vi "Database Message Loop.vi"(8 "error in":errorcluster, 10 "Message Queues":T1, 11 "Clust Refnum":refnum<vi>) -> (0 "error out":errorcluster)   [LabVIEW 2025]
doc: "This example allows you to perform several tasks on the specified table in a database named LabVIEW.mdb located in the LabVIEW examples>>database directory.\n\nThis VI is running when you open it. Select one of the tabs and enter the appropriate data. Press the Go button to complete the displayed tab option.\n\nAutomatic - This option inserts a new record into the specified table. The record is specified by a cluster containing the correct number of elements and of the data types defined by the specified table. \n\nSQL Query - This option performs the specified SQL query.\n\nParameterized SQL Query - This option performs the specified SQL query as a parameterized SQL Query. This method is faster and more efficient than directly executing an SQL query because it sets up all the parameters prior to doing the command."
uses:
  support/Message Queue/All Message Queues.ctl
  support/Message Queue/Message Cluster.ctl
  controls/Design_Results.ctl
  <vilib>/drjdpowell/SQLite Library/SQL Statement/SQL Statement.lvclass
  <vilib>/drjdpowell/SQLite Library/SQL Connection/Connection.lvclass
  <vilib>/drjdpowell/SQLite Library/SQL Statement/SQL Statement.lvclass/SQL Statement.ctl
  <vilib>/drjdpowell/SQLite Library/SQL Connection/Open (string).vi
  <vilib>/drjdpowell/SQLite Library/SQL Statement/Bind Timestamp (Local Time Offset).vi
  <vilib>/drjdpowell/SQLite Library/SQL Statement/Bind Real.vi
  <vilib>/drjdpowell/SQLite Library/SQL Statement/Bind Text.vi
  <vilib>/drjdpowell/SQLite Library/SQL Statement/Bind Integer.vi
  <vilib>/drjdpowell/SQLite Library/SQL Statement/Step.vi
  <vilib>/JDP Science/JDP Science Common Utilities/Timestamp/Timestamp to Text.vi
  <vilib>/drjdpowell/SQLite Library/SQL Statement/Bind UTF-8 Text.vi
  <vilib>/Utility/error.llb/Error Cluster From Error Code.vi
  <vilib>/drjdpowell/SQLite Library/SQL Connection/Execute SQL (No results).vi
  <vilib>/drjdpowell/SQLite Library/SQL Statement/Error Message.vi
  <vilib>/ErrorRing/Error Ring.xnode
  support/Message Queue/Message Queue.lvlib
  <vilib>/drjdpowell/SQLite Library/SQLite.lvlib
panel:
  # "Simulator Fit"
  # "Empirical Fit"
  # "="
  # "P"
  # "* X"
  # "P"
  # "="
  # "* X"
  # "drop"
  # "drop"
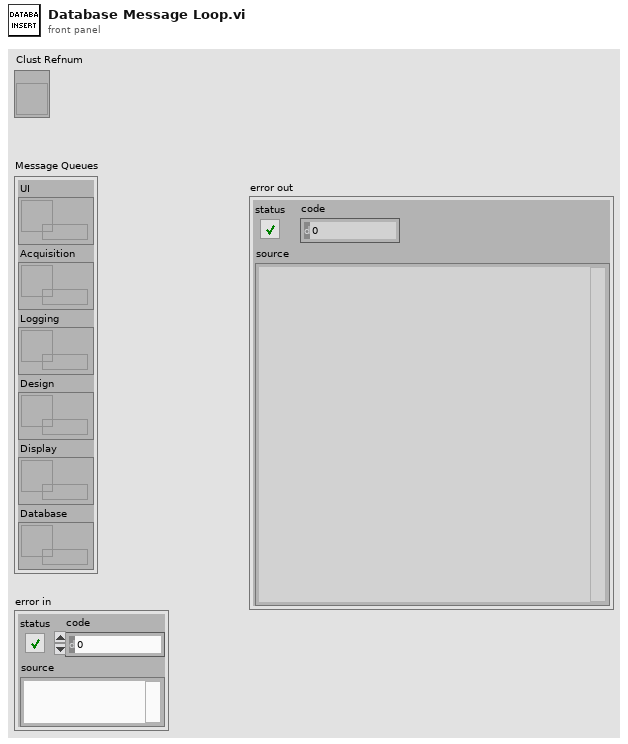
[diagram p1: front panel]
types:
  T1 = typedef "Message Queue.lvlib/All Message Queues.ctl" = cluster{"UI":refnum<queue>, "Acquisition":refnum<queue>, "Logging":refnum<queue>, "Design":refnum<queue>, "Display":refnum<queue>, "Database":refnum<queue>}
  T2 = typedef "Results.ctl" = cluster{"Design Results":cluster{"Model Validation: Simulated vs. Empirical Airflow Data":cluster{dbl[], dbl[]}[], "Amplitude - Empirical":string, "Power - Empirical":string, "Amplitude - Sim":string, "Power - Sim":string, "Flow Type":u32, "Optimized Inlet \nOrifice Diameter (in)":dbl, "Flow Type Name":string}}
  T3 = cluster{"Model Validation: Simulated vs. Empirical Airflow Data[0]":cluster{dbl[], dbl[]}, "Model Validation: Simulated vs. Empirical Airflow Data[1]":cluster{dbl[], dbl[]}, "Model Validation: Simulated vs. Empirical Airflow Data[2]":cluster{dbl[], dbl[]}, "Model Validation: Simulated vs. Empirical Airflow Data[3]":cluster{dbl[], dbl[]}, "Model Validation: Simulated vs. Empirical Airflow Data[4]":cluster{dbl[], dbl[]}, "Model Validation: Simulated vs. Empirical Airflow Data[5]":cluster{dbl[], dbl[]}, "Model Validation: Simulated vs. Empirical Airflow Data[6]":cluster{dbl[], dbl[]}, "Model Validation: Simulated vs. Empirical Airflow Data[7]":cluster{dbl[], dbl[]}, "Model Validation: Simulated vs. Empirical Airflow Data[8]":cluster{dbl[], dbl[]}}
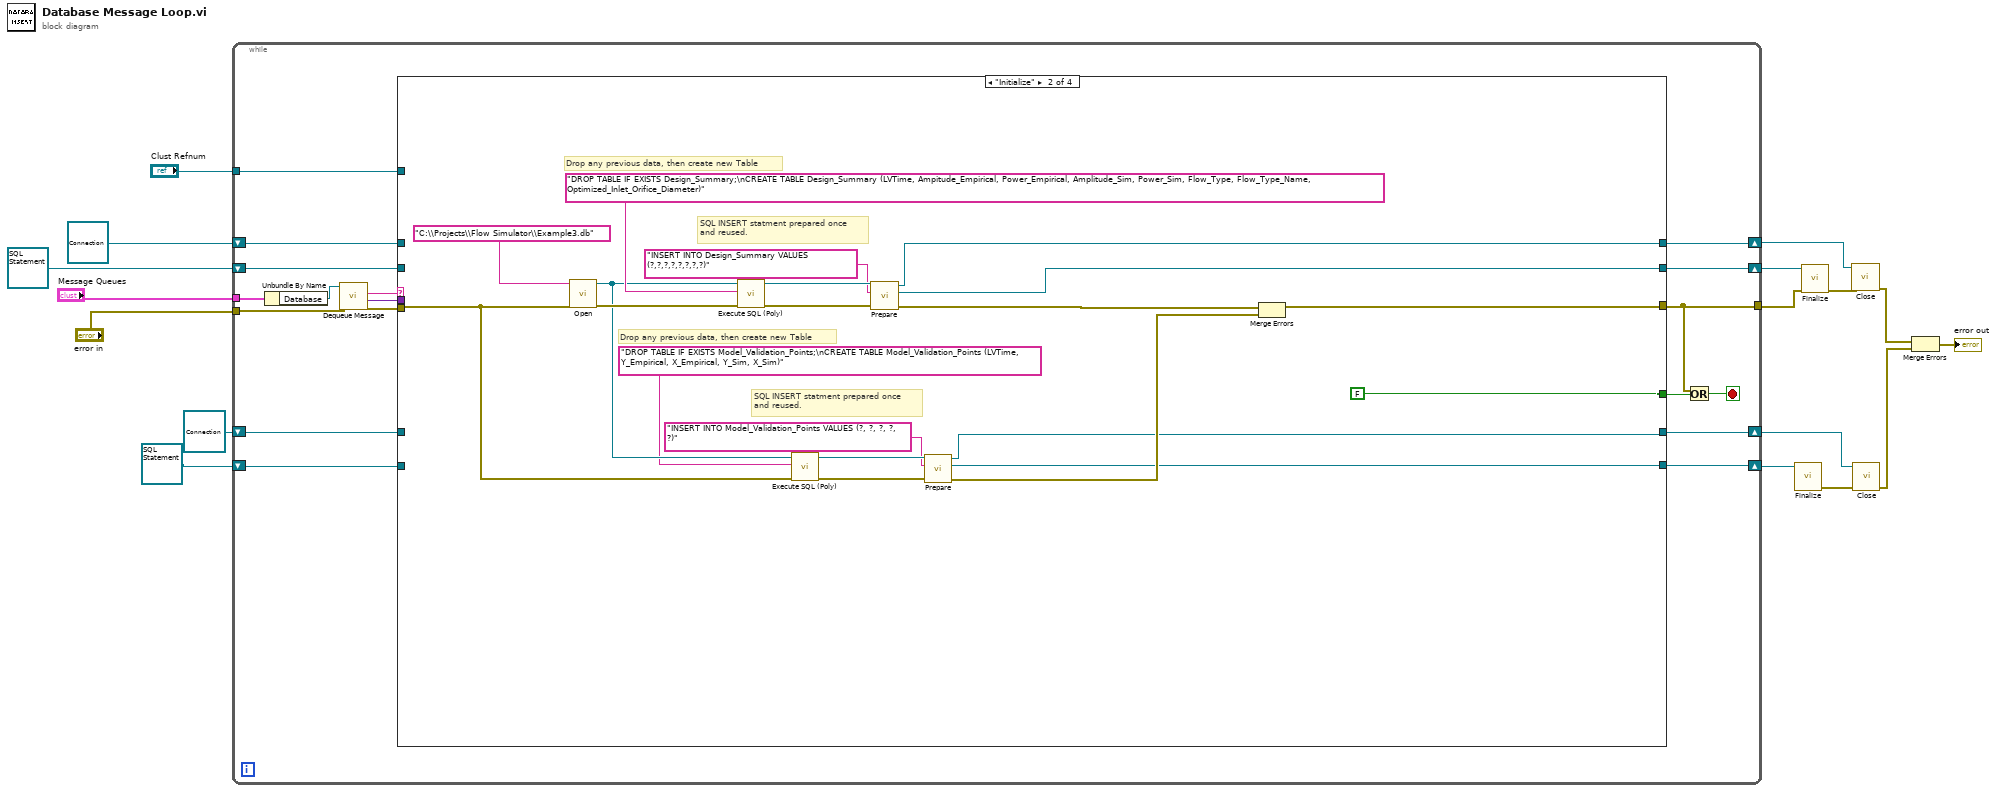
[diagram p0: block diagram]
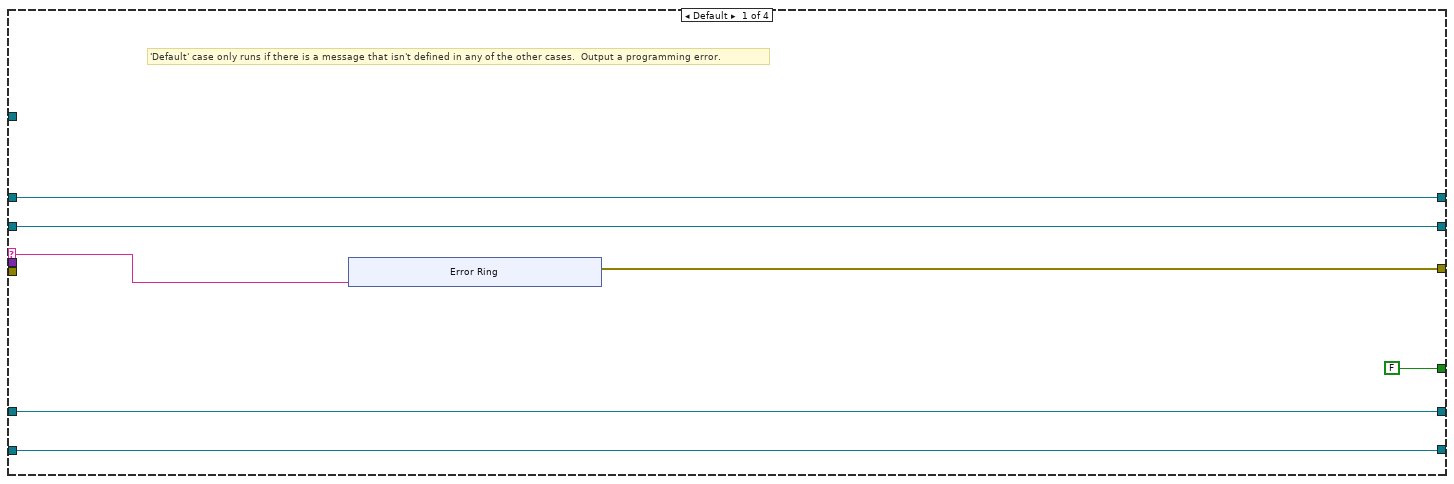
[diagram p2: hidden frame]
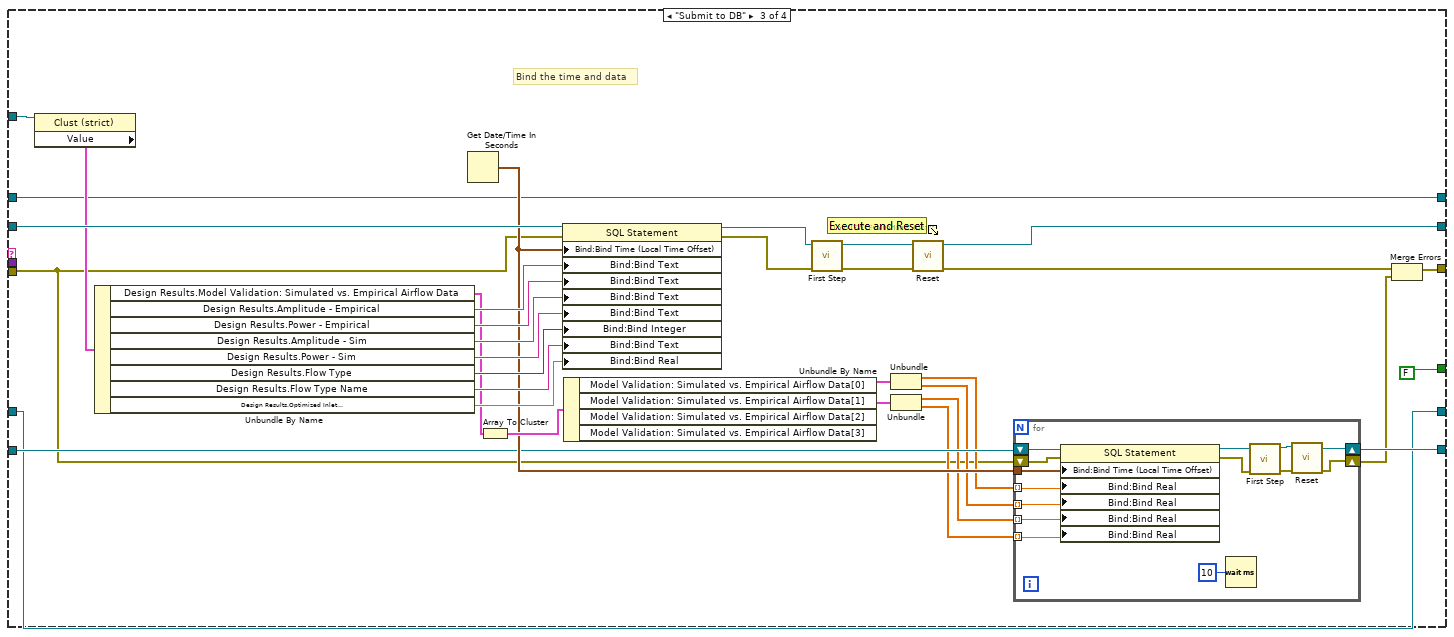
[diagram p3: hidden frame]
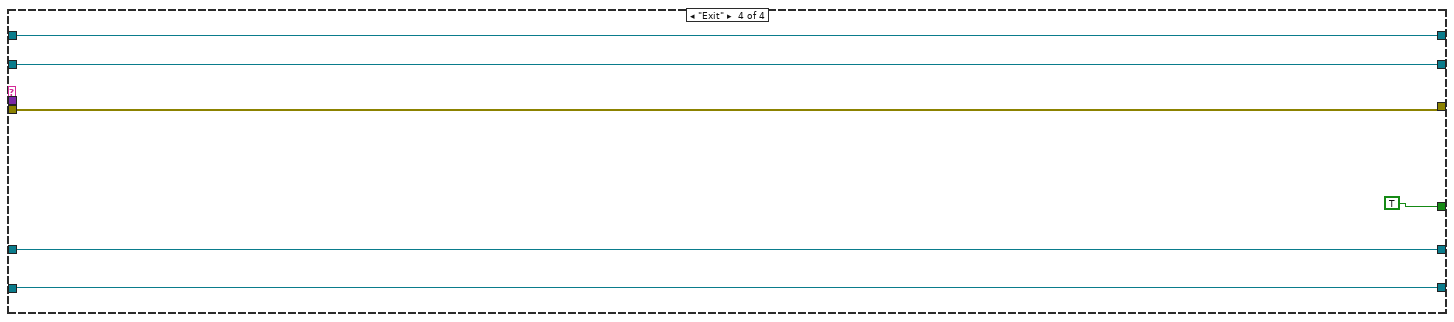
[diagram p4: hidden frame]
diagram:
  n1 = while {
    tunnel: "Message Queues" -> [w34]
    tunnel: [w30] -> w8
    tunnel: "error in" -> [w31]
    shift-right: [w26] -> w9
    shift-left: refnum<class "SQL Statement.lvclass"> refnum ("SQL Statement") -> [w27]
    shift-right: [w23] -> w12
    shift-left: refnum<class "SQL Statement.lvclass"> refnum ("SQL Statement") -> [w22]
    tunnel: "Clust Refnum" -> [w24]
    shift-right: [w21] -> w10
    shift-left: refnum<class "Connection.lvclass"> refnum ("SQLite Connection") -> [w19]
    shift-right: [w20] -> w6
    shift-left: refnum<class "Connection.lvclass"> refnum ("SQLite Connection") -> [w18]
    stop <- w28 stop-if-true
    n2 = Unbundle By Name(w34) -> ("Database"=w33:refnum<queue>)
    n3 = call "Dequeue Message.vi"("error in (no error)"=w31, "Message Queue"=w33) -> ("error out"=w32:errorcluster, "Message Data"=w25:variant, "Message"=w35:string)  [unwired: 6 in, 1 out]
    n4 = case shown="\"Initialize\"" w35 {
      selector: w35 -> [w40 _ _ _]
      tunnel: [FALSE FALSE FALSE TRUE] -> w29
      tunnel: [w41 w53 w70 w121] -> w30
      tunnel: w32 -> [_ w55 w76 w121]
      tunnel: [w39 w62 w100 w120] -> w26
      tunnel: w27 -> [w39 _ w88 w120]
      tunnel: w25 -> [_ _ _ _]
      tunnel: [w38 w52 w75 w119] -> w23
      tunnel: w22 -> [w38 _ w83 w119]
      tunnel: w24 -> [_ _ w89 _]
      tunnel: [w37 w51 w74 w118] -> w21
      tunnel: [w36 w50 w73 w117] -> w20
      tunnel: w19 -> [w37 _ w74 w118]
      tunnel: w18 -> [w36 _ w73 w117]
      frame Default {
        # "'Default' case only runs if there is a message that isn't defined in any of the other cases.  Output a programming error."
        n5 = xnode "Error Ring"("parameter 0"=w40) -> ("error out"=w41:errorcluster)
      }
      frame "Initialize" {
        # "SQL INSERT statment prepared once\nand reused."
        # "Drop any previous data, then create new Table"
        # "SQL INSERT statment prepared once\nand reused."
        # "Drop any previous data, then create new Table"
        n6 = call-poly <vilib>:"Open.vi"("error in (no error)"=w55, "db file"="C:\\Projects\\Flow Simulator\\Example3.db") -> ("error out"=w68:errorcluster, "SQLite Connection"=w58:refnum<class "Connection.lvclass">)  [unwired: 8 in]
        n7 = call-poly <vilib>:"Execute SQL (Poly).vi"("error in (no error)"=w68, "SQL"="DROP TABLE IF EXISTS Design_Summary;\nCREATE TABLE Design_Summary (LVTime, Ampitude_Empirical, Power_Empirical, Amplitude_Sim, Power_Sim, Flow_Type, Flow_Type_Name, Optimized_Inlet_Orifice_Diameter)", "SQLite Connection in"=w58) -> ("error out"=w66:errorcluster, "SQLite Connection"=w65:refnum<class "Connection.lvclass">)  [unwired: 7 in]
        n8 = call-poly <vilib>:"Execute SQL (Poly).vi"("error in (no error)"=w55, "SQL"="DROP TABLE IF EXISTS Model_Validation_Points;\nCREATE TABLE Model_Validation_Points (LVTime, Y_Empirical, X_Empirical, Y_Sim, X_Sim)", "SQLite Connection in"=w58) -> ("error out"=w61:errorcluster, "SQLite Connection"=w60:refnum<class "Connection.lvclass">)  [unwired: 7 in]
        n9 = call <vilib>:"Prepare.vi"("error in (no error)"=w66, "SQL"="INSERT INTO Design_Summary VALUES (?,?,?,?,?,?,?,?)", "SQLite Connection in"=w65) -> ("error out"=w54:errorcluster, "SQL Statement"=w62:refnum<class "SQL Statement.lvclass">, "SQLite Connection"=w51:refnum<class "Connection.lvclass">)  [unwired: 4 in, 2 out]
        n10 = call <vilib>:"Prepare.vi"("error in (no error)"=w61, "SQL"="INSERT INTO Model_Validation_Points VALUES (?, ?, ?, ?, ?)", "SQLite Connection in"=w60) -> ("error out"=w56:errorcluster, "SQL Statement"=w52:refnum<class "SQL Statement.lvclass">, "SQLite Connection"=w50:refnum<class "Connection.lvclass">)  [unwired: 4 in, 2 out]
        n11 = Merge Errors(w54, w56) -> (w53:errorcluster)
      }
      frame "Submit to DB" {
        # "Bind the time and data"
        n12 = property class="Clust (strict)"(reference=w89) -> ("Value"=w87:T2)  [unwired: 1 in, 2 out]
        n13 = Unbundle By Name(w87) -> ("Design Results.Model Validation: Simulated vs. Empirical Airflow Data"=w86:cluster{dbl[], dbl[]}[], "Design Results.Amplitude - Empirical"=w97:string, "Design Results.Power - Empirical"=w96:string, "Design Results.Amplitude - Sim"=w95:string, "Design Results.Power - Sim"=w94:string, "Design Results.Flow Type"=w93:u32, "Design Results.Flow Type Name"=w92:string, "Design Results.Optimized Inlet \nOrifice Diameter (in)"=w91:dbl)
        n14 = Get Date/Time In Seconds() -> (seconds since 1Jan1904=w84:timestamp)
        n15 = Array To Cluster(array=w86) -> (cluster=w85:T3)
        n16 = property class="SQL Statement"(reference=w88, error in=w76, "Bind:Bind Time (Local Time Offset)"=w84, "Bind:Bind Text"=w97, "Bind:Bind Text"=w96, "Bind:Bind Text"=w95, "Bind:Bind Text"=w94, "Bind:Bind Integer"=w93, "Bind:Bind Text"=w92, "Bind:Bind Real"=w91) -> (reference out=w90:refnum<class "SQL Statement.lvclass">, error out=w98:errorcluster)
        n17 = Unbundle By Name(w85) -> ("Model Validation: Simulated vs. Empirical Airflow Data[0]"=w82:cluster{dbl[], dbl[]}, "Model Validation: Simulated vs. Empirical Airflow Data[1]"=w79:cluster{dbl[], dbl[]})  [unwired: 2 out]
        n18 = call <vilib>:"First Step.vi"("error in (no error)"=w98, "SQL Statement in"=w90) -> ("error out"=w101:errorcluster, "SQL Statement"=w99:refnum<class "SQL Statement.lvclass">)  [unwired: 7 in, 1 out]
        n19 = Unbundle(w82) -> (w81:dbl[], w80:dbl[])
        n20 = Unbundle(w79) -> (w78:dbl[], w77:dbl[])
        n21 = call <vilib>:"Reset.vi"("error in (no error)"=w101, "SQL Statement in"=w99) -> ("error out"=w72:errorcluster, "SQL Statement"=w100:refnum<class "SQL Statement.lvclass">)  [unwired: 8 in]
        n22 = for {
          tunnel: w84 -> [w116]
          tunnel: w81 -> [w114] mode=indexing
          tunnel: w80 -> [w113] mode=indexing
          tunnel: w78 -> [w112] mode=indexing
          tunnel: w77 -> [w111] mode=indexing
          shift-right: [w104] -> w71
          shift-left: w76 -> [w105]
          shift-right: [w106] -> w75
          shift-left: w83 -> [w115]
          n23 = property class="SQL Statement"(reference=w115, error in=w105, "Bind:Bind Time (Local Time Offset)"=w116, "Bind:Bind Real"=w114, "Bind:Bind Real"=w113, "Bind:Bind Real"=w112, "Bind:Bind Real"=w111) -> (reference out=w108:refnum<class "SQL Statement.lvclass">, error out=w107:errorcluster)
          n24 = Wait (ms)(milliseconds to wait=u32 10) -> ()  [unwired: 1 out]
          n25 = call <vilib>:"First Step.vi"("error in (no error)"=w107, "SQL Statement in"=w108) -> ("error out"=w110:errorcluster, "SQL Statement"=w109:refnum<class "SQL Statement.lvclass">)  [unwired: 7 in, 1 out]
          n26 = call <vilib>:"Reset.vi"("error in (no error)"=w110, "SQL Statement in"=w109) -> ("error out"=w104:errorcluster, "SQL Statement"=w106:refnum<class "SQL Statement.lvclass">)  [unwired: 8 in]
        }
        n27 = Merge Errors(w72, w71) -> (w70:errorcluster)
      }
      frame "Exit" {
      }
    }
    n28 = Or(x=w30, y=w29) -> (x .or. y?=w28:bool)
  }
  n29 = call <vilib>:"Finalize.vi"("SQL Statement in"=w12) -> ("error out"=w11:errorcluster)  [unwired: 10 in]
  n30 = call <vilib>:"Finalize.vi"("error in (no error)"=w8, "SQL Statement in"=w9) -> ("error out"=w7:errorcluster)  [unwired: 9 in]
  n31 = call-dynamic "Close.vi"("error in (no error)"=w7, "SQLite Connection in"=w10) -> ("error out"=w5:errorcluster)  [unwired: 9 in]
  n32 = call-dynamic "Close.vi"("error in (no error)"=w11, "SQLite Connection in"=w6) -> ("error out"=w4:errorcluster)  [unwired: 9 in]
  n33 = Merge Errors(w5, w4) -> (→"error out":errorcluster)
